vi "micro_Devices.vi"() -> ()   [LabVIEW 2014]
doc: "André Romero - 2023\nandretec@ifsc.usp.br\nIFSC - USP"
uses:
  Controller.ctl
  Thorlabs-Vector-Move/aptTec/Thorlabs-V2/Global Motors.vi
panel:
  out "Z ini":dbl
  out "Array Structures Ind":refnum<vi>[](array[refnum])
  in  "Tab Control":T1(tab)=enum."Cubes"
  in  "start-stop":bool
  in  "step size (mm)":dbl=10.0
  in  "Min   Z":bool
  in  "Max  Z":bool
  in  "Min":bool
  in  "Max":bool
  in  "Z (m/s)":dbl=50.0
  in  "XY (m/s)":dbl format="%#_5g"
  out "Motor Y":bool=TRUE
  out "Motor X":bool=TRUE
  out "Motor Z":bool=TRUE
  in  "Motor - Z":refnum<k7>(container)
  in  "Motor - Y":refnum<k7>(container)
  in  "Motor - X":refnum<k7>(container)
  out "current cube":i32
  out "current Layer":i32=1
  out "Total Progress (%)":u8(slide) caption="Layer Progress (%)" scale=0.0..25.0
  out "Layer Progress (%)":u8(slide)=100 scale=0.0..100.0
  in  "Line step size (mm)":dbl=1.0
  out "Lines Progress (%)":u8(slide)=42 scale=0.0..100.0
  in  "Stop Button":bool
  in  "Go Cubes":bool
  in  "Array of Structures":bool
  in  "Velocity (m/s)":dbl=50.0
  out "Layers":dbl=1.0
  in  "Delta Y (um)":dbl=50.0
  in  "Delta X (um)":dbl=50.0
  in  "Number of Lines":i32=2
  in  "Number of Columns":i32=5
  in  "Layer height (mm)":dbl=1.0
  in  "Height (mm)":dbl=1.0
  in  "Length (mm)":dbl=20.0
  in  "Width (mm)":dbl=20.0
  out "X ini":dbl
  out "Y ini":dbl
  in  "Initial position Z":bool=TRUE
  in  "Z offset (mm)":dbl=10.0
  in  "Z offset":bool
  in  "Motor - Z2":refnum<k7>(container)
  out "XY Graph":cluster{dbl[], dbl[]}(graph)
  in  "Go Test":bool
  in  "Density points":i32
  # "Velocity"
  # "Jog"
  # "mm"
  # "Z"
  # "Settings"
  # "Control"
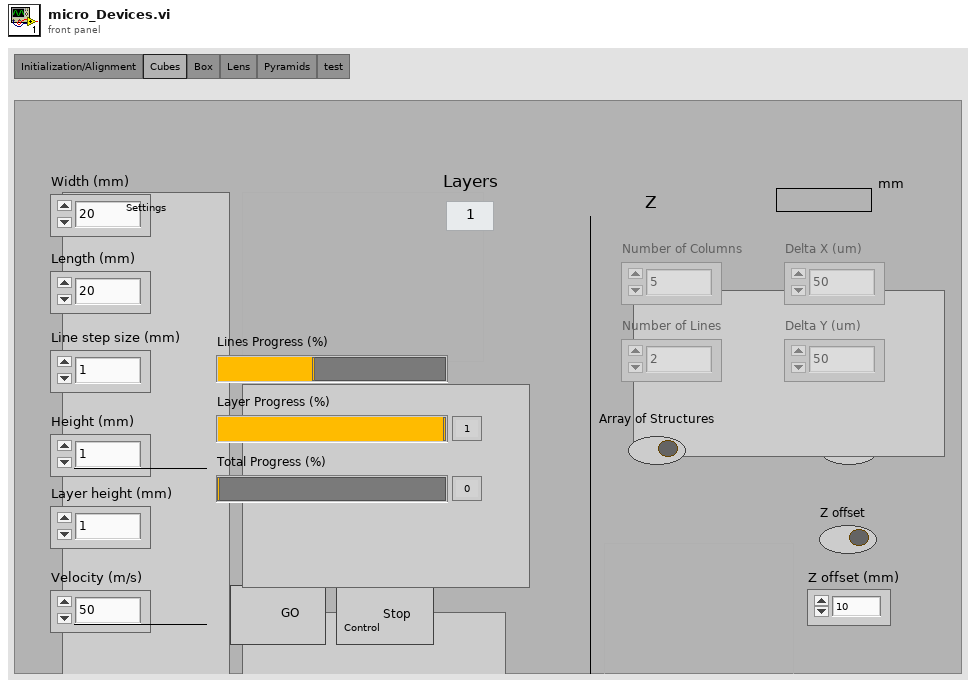
[diagram p1: front panel]
types:
  T1 = enum32{"Initialization/Alignment", "Cubes", "Box", "Lens", "Pyramids", "test"}
  T2 = typedef "Controller.ctl" = enum16{"Initialize", "Wait for Event", "Cubes", "Lens", "Box", "test tap"}
  T3 = typedef "eventvkey.ctl" = enum16{"ASCII", "Enter", "Return", "Shift", "Ctrl", "Alt", "Cmd", "Opt", "Caps", "NumLock", "Clear", "Break", "Up", "Down", "Left", "Right", "Insert", "Delete", "Home", "End", "PageUp", "PageDown", "Escape", "Help", "Pause", "ScrollLock", "F1", "F2", "F3", "F4", "F5", "F6", "F7", "F8", "F9", "F10", "F11", "F12", "F13", "F14", "F15", "F16", "F17", "F18", "F19", "F20", "F21", "F22", "F23", "F24", "Play", "VolumeUp", "VolumeDown", "Mute", "Two Byte Char"}
  T4 = enum8{"Enabled", "Disabled", "Disabled and Grayed Out"}
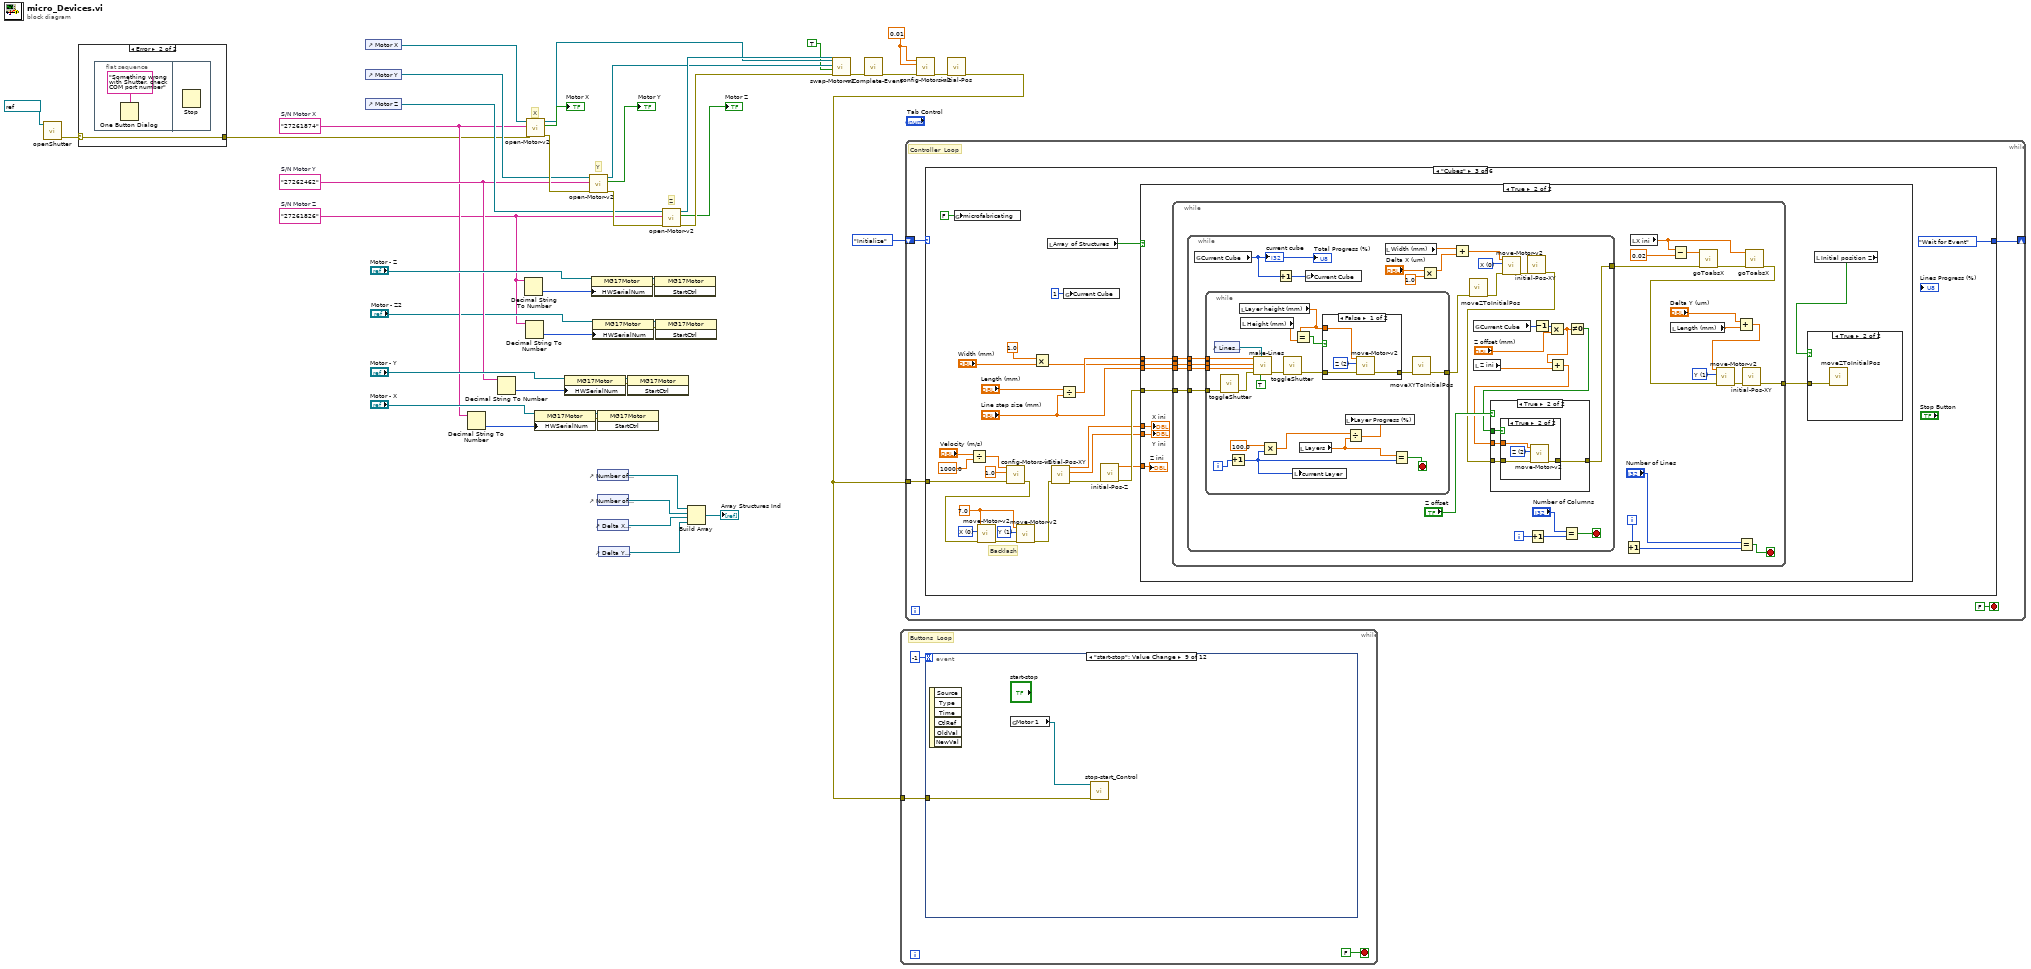
[diagram p0: block diagram]
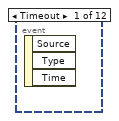
[diagram p3: hidden frame]
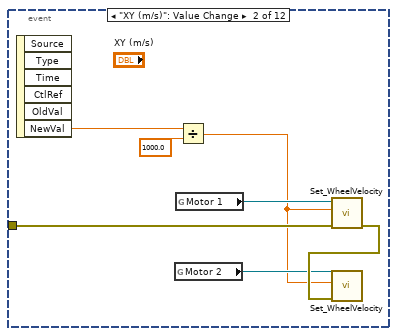
[diagram p4: hidden frame]
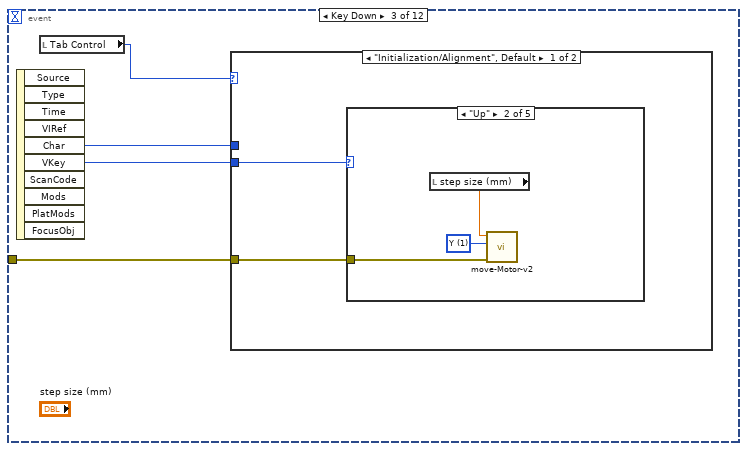
[diagram p5: hidden frame]
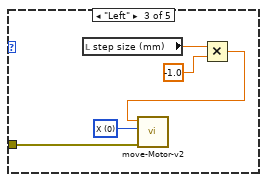
[diagram p7: hidden frame]
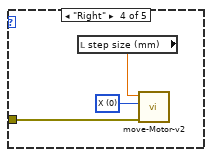
[diagram p8: hidden frame]
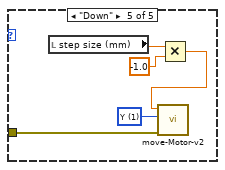
[diagram p9: hidden frame]
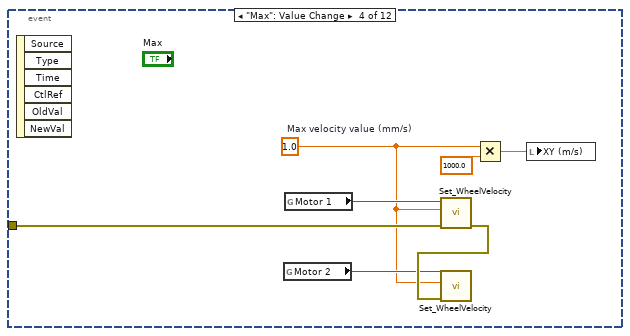
[diagram p11: hidden frame]
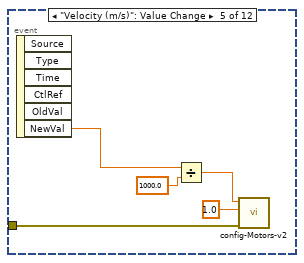
[diagram p12: hidden frame]
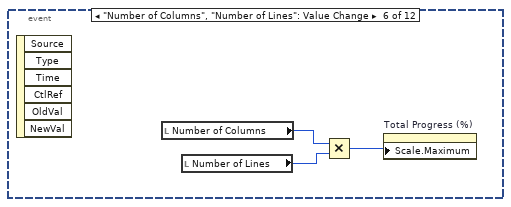
[diagram p13: hidden frame]
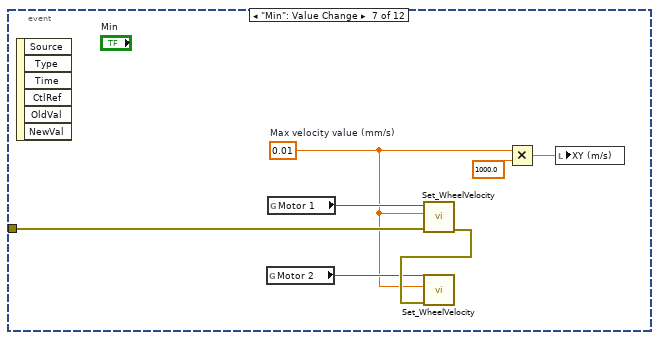
[diagram p14: hidden frame]
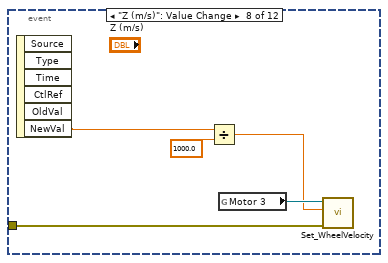
[diagram p15: hidden frame]
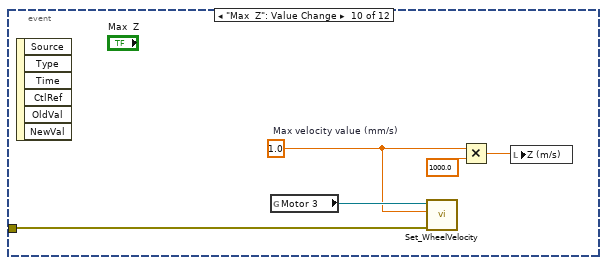
[diagram p16: hidden frame]
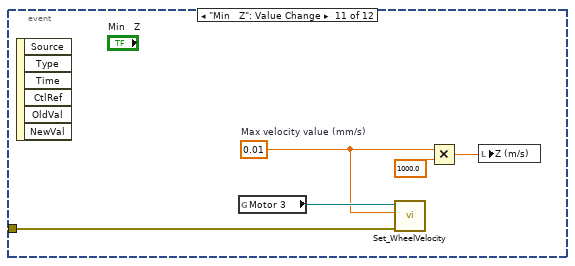
[diagram p17: hidden frame]
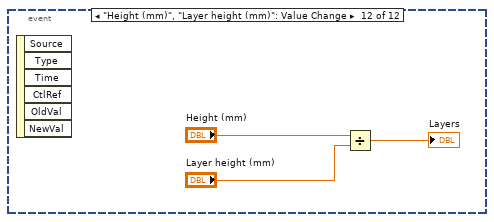
[diagram p18: hidden frame]
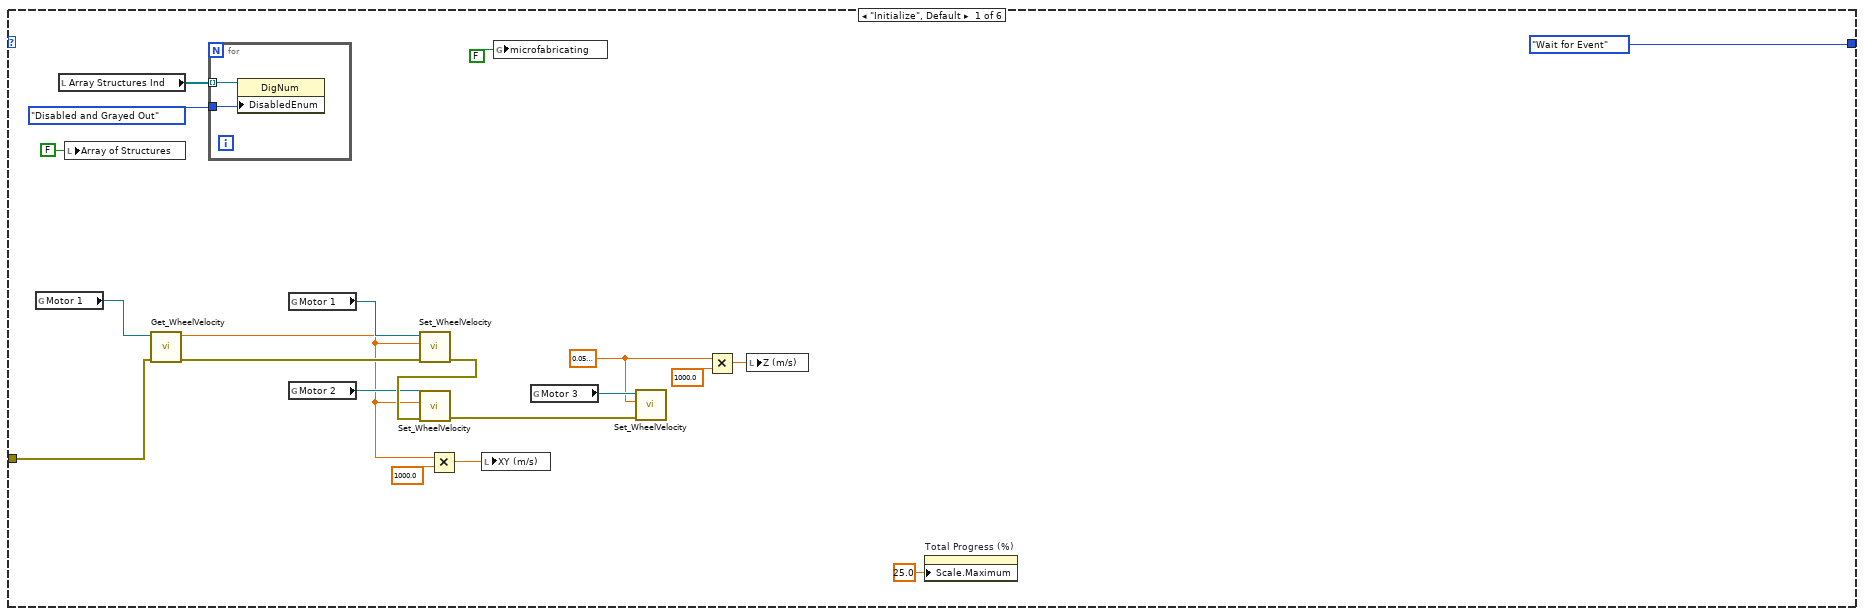
[diagram p19: hidden frame]
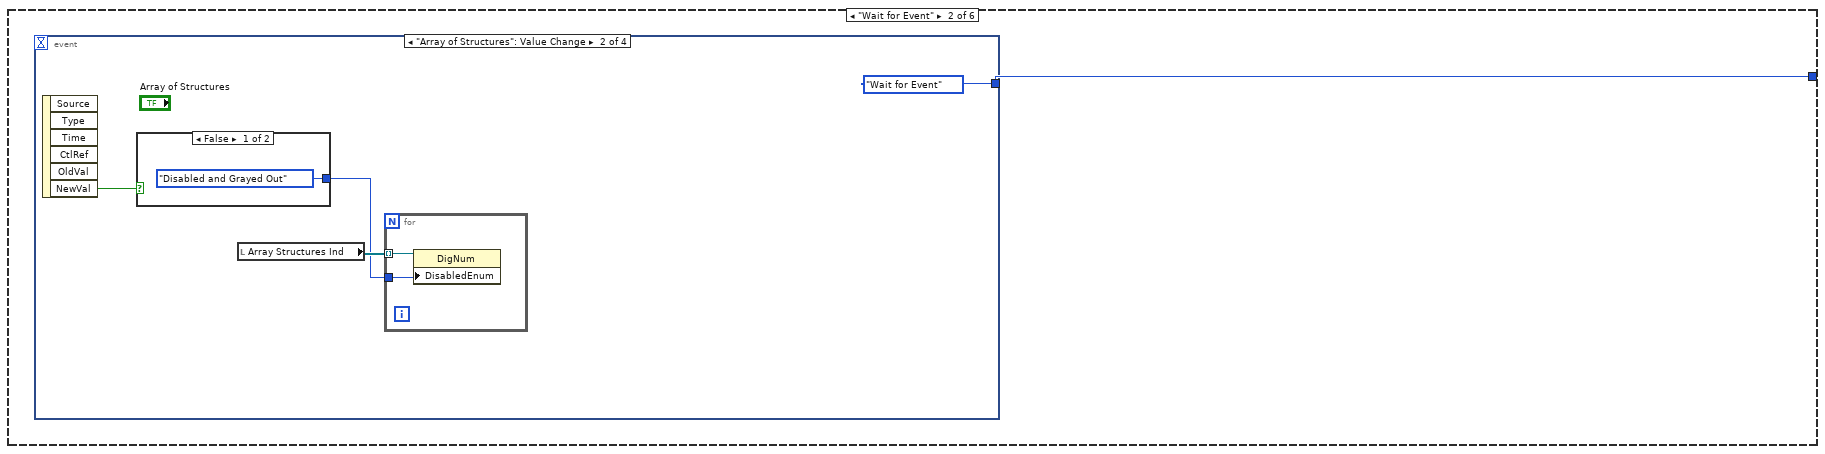
[diagram p20: hidden frame]
diagram:
  w29 = 0.01 ("Acc")
  w16 = "27262462"  # S/N Motor Y
  w15 = "27261874"  # S/N Motor X
  w1 = "27261826"  # S/N Motor Z
  # "X"
  # "Y"
  # "Z"
  n1 = call "openShutter.vi"("VISA Refnum in"=refnum<visa-resource-name> "COM3") -> ("error out"=w7:errorcluster)  [unwired: 9 in, 1 out]
  n2 = case shown="Error" w7 {
    selector: w7 -> [w47 w48]
    tunnel: [w47 w48] -> w6
    frame No Error {
    }
    frame Error {
      n3 = flat-sequence {
        frame #0 {
          n4 = One Button Dialog(message="Something wrong with Shutter, check COM port number") -> ()  [unwired: 1 in, 1 out]
        }
        frame #1 {
          n5 = Stop() -> ()  [unwired: 1 in]
        }
      }
    }
  }
  n6 = control-ref of="Motor X"() -> (w43:refnum<vi>)
  n7 = control-ref of="Motor Y"() -> (w42:refnum<vi>)
  n8 = control-ref of="Motor Z"() -> (w38:refnum<vi>)
  n9 = Decimal String To Number(string=w15) -> (number=w17:i32)  [unwired: 2 in, 1 out]
  n10 = Decimal String To Number(string=w16) -> (number=w21:i32)  [unwired: 2 in, 1 out]
  n11 = Decimal String To Number(string=w1) -> (number=w25:i32)  [unwired: 2 in, 1 out]
  n12 = Decimal String To Number(string=w1) -> (number=w2:i32)  [unwired: 2 in, 1 out]
  n13 = call "open-Motor-v2.vi"("Error In"=w6, "S/N Motor"=w15, "ref Boolean in"=w43) -> ("Error Out"=w46:errorcluster, "Motor Status"=→"Motor X":bool, "Refnum out"=w11:refnum<k7>)  [unwired: 6 in]
  n14 = property class="MG17Motor"(reference="Motor - X", "HWSerialNum"=w17) -> (reference out=w18:refnum<k7>, error out=w19:errorcluster)  [unwired: 1 in]
  n15 = property class="MG17Motor"(reference="Motor - Y", "HWSerialNum"=w21) -> (reference out=w22:refnum<k7>, error out=w23:errorcluster)  [unwired: 1 in]
  n16 = call "open-Motor-v2.vi"("Error In"=w46, "S/N Motor"=w16, "ref Boolean in"=w42) -> ("Error Out"=w40:errorcluster, "Motor Status"=→"Motor Y":bool, "Refnum out"=w10:refnum<k7>)  [unwired: 6 in]
  n17 = property class="MG17Motor"(reference="Motor - Z", "HWSerialNum"=w25) -> (reference out=w26:refnum<k7>, error out=w27:errorcluster)  [unwired: 1 in]
  n18 = property class="MG17Motor"(reference="Motor - Z2", "HWSerialNum"=w2) -> (reference out=w3:refnum<k7>, error out=w4:errorcluster)  [unwired: 1 in]
  n19 = invoke class="MG17Motor" method="StartCtrl"(reference=w18, error in=w19) -> ()  [unwired: 1 in, 3 out]
  n20 = control-ref of="Number of Lines"() -> (w34:refnum<vi>)
  n21 = control-ref of="Number of Columns"() -> (w33:refnum<vi>)
  n22 = control-ref of="Delta X (um)"() -> (w32:refnum<vi>)
  n23 = control-ref of="Delta Y (um)"() -> (w31:refnum<vi>)
  n24 = invoke class="MG17Motor" method="StartCtrl"(reference=w22, error in=w23) -> ()  [unwired: 1 in, 3 out]
  n25 = invoke class="MG17Motor" method="StartCtrl"(reference=w26, error in=w27) -> ()  [unwired: 1 in, 3 out]
  n26 = invoke class="MG17Motor" method="StartCtrl"(reference=w3, error in=w4) -> ()  [unwired: 1 in, 3 out]
  n27 = call "open-Motor-v2.vi"("Error In"=w40, "S/N Motor"=w1, "ref Boolean in"=w38) -> ("Error Out"=w39:errorcluster, "Motor Status"=→"Motor Z":bool, "Refnum out"=w36:refnum<k7>)  [unwired: 6 in]
  n28 = Build Array(w34, w33, w32, w31) -> (→"Array Structures Ind":refnum<vi>[])
  n29 = call "swap-Motor-v2.vi"("Refnum in M3"=w36, "error in (no error)"=w39, "Swap motor"=TRUE, "Refnum in M2"=w10, "Refnum in M1"=w11) -> ("error out"=w14:errorcluster)  [unwired: 6 in]
  n30 = call "mComplete-Event.vi"("Error In"=w14) -> ("Error Out"=w13:errorcluster)  [unwired: 10 in]
  n31 = call "config-Motors-v2.vi"("error in"=w13, "Acc"=w29, "Velocity"=w29) -> ("error out"=w41:errorcluster)  [unwired: 8 in]
  n32 = call "initial-Pos.vi"("error in (no error)"=w41) -> ("error out"=w12:errorcluster)  [unwired: 10 in]
  n33 = while {
    tunnel: w12 -> [w51]
    stop <- FALSE stop-if-true
    # "Buttons  Loop"
    n34 = event shown="[8] \"start-stop\": Value Change" {
      selector: _ -> [_ _ _ _ _ _ _ _ _ _ _ _]
      dyn-events: _ -> [_ _ _ _ _ _ _ _ _ _ _ _]
      timeout: -1 -> [_ _ _ _ _ _ _ _ _ _ _ _]
      tunnel: w51 -> [_ w58 w60 w85 w89 _ w100 w104 w110 w111 w116 _]
      event Timeout {
        n35 = event-data() -> ()  [unwired: 1 in, 3 out]
      }
      event "XY (m/s)": Value Change {
        n36 = event-data() -> ("NewVal"=w55:dbl)  [unwired: 1 in, 5 out]
        n37 = global read "Global Motors.vi" "Motor 2"() -> (w56:refnum<k7>)
        n38 = global read "Global Motors.vi" "Motor 1"() -> (w59:refnum<k7>)
        n39 = Divide(x=w55, y=1000.0) -> (x/y=w54:dbl)
        n40 = call "Set_WheelVelocity.vi"("error in"=w58, "fWheelVel"=w54, "MG17Motor in"=w59) -> ("error out"=w57:errorcluster)  [unwired: 8 in]
        n41 = call "Set_WheelVelocity.vi"("error in"=w57, "fWheelVel"=w54, "MG17Motor in"=w56) -> ()  [unwired: 8 in, 1 out]
      }
      event Key Down {
        n42 = event-data() -> ("Char"=w62:i16, "VKey"=w61:T3)  [unwired: 1 in, 8 out]
        n43 = local read "Tab Control"() -> (w63:T1)
        n44 = case shown="\"Initialization/Alignment\", Default" w63 {
          tunnel: w62 -> [_ _]
          tunnel: w61 -> [w65 _]
          tunnel: w60 -> [w64 _]
          frame "Initialization/Alignment", Default {
            n45 = case shown="\"Up\"" w65 {
              tunnel: w64 -> [_ w68 w73 w76 w80]
              frame "ASCII", Default {
              }
              frame "Up" {
                w67 = u16 1 items=["X", "Y", "Z"] ("Axis")
                n46 = local read "step size (mm)"() -> (w66:dbl)
                n47 = call "move-Motor-v2.vi"("error in"=w68, "Axis"=w67, "Distance (um)"=w66) -> ()  [unwired: 8 in, 1 out]
              }
              frame "Left" {
                w72 = u16 0 items=["X", "Y", "Z"] ("Axis")
                n48 = local read "step size (mm)"() -> (w71:dbl)
                n49 = Multiply(x=w71, y=-1.0) -> (x*y=w69:dbl)
                n50 = call "move-Motor-v2.vi"("error in"=w73, "Axis"=w72, "Distance (um)"=w69) -> ()  [unwired: 8 in, 1 out]
              }
              frame "Right" {
                w75 = u16 0 items=["X", "Y", "Z"] ("Axis")
                n51 = local read "step size (mm)"() -> (w74:dbl)
                n52 = call "move-Motor-v2.vi"("error in"=w76, "Axis"=w75, "Distance (um)"=w74) -> ()  [unwired: 8 in, 1 out]
              }
              frame "Down" {
                w81 = u16 1 items=["X", "Y", "Z"] ("Axis")
                n53 = local read "step size (mm)"() -> (w79:dbl)
                n54 = Multiply(x=w79, y=-1.0) -> (x*y=w77:dbl)
                n55 = call "move-Motor-v2.vi"("error in"=w80, "Axis"=w81, "Distance (um)"=w77) -> ()  [unwired: 8 in, 1 out]
              }
            }
          }
          frame "Cubes" {
          }
        }
      }
      event "Max": Value Change {
        w83 = 1.0  # Max velocity value (mm/s)
        n56 = event-data() -> ()  [unwired: 1 in, 6 out]
        n57 = global read "Global Motors.vi" "Motor 2"() -> (w86:refnum<k7>)
        n58 = global read "Global Motors.vi" "Motor 1"() -> (w88:refnum<k7>)
        n59 = call "Set_WheelVelocity.vi"("error in"=w85, "fWheelVel"=w83, "MG17Motor in"=w88) -> ("error out"=w87:errorcluster)  [unwired: 8 in]
        n60 = call "Set_WheelVelocity.vi"("error in"=w87, "fWheelVel"=w83, "MG17Motor in"=w86) -> ()  [unwired: 8 in, 1 out]
        n61 = Multiply(x=w83, y=1000.0) -> (x*y=w82:dbl)
        n62 = local write "XY (m/s)"(w82) -> ()
      }
      event "Velocity (m/s)": Value Change {
        n63 = event-data() -> ("NewVal"=w93:dbl)  [unwired: 1 in, 5 out]
        n64 = Divide(x=w93, y=1000.0) -> (x/y=w91:dbl)
        n65 = call "config-Motors-v2.vi"("error in"=w89, "Acc"=1.0, "Velocity"=w91) -> ()  [unwired: 8 in, 1 out]
      }
      event "Number of Columns", "Number of Lines": Value Change {
        n66 = event-data() -> ()  [unwired: 1 in, 6 out]
        n67 = local read "Number of Columns"() -> (w95:i32)
        n68 = local read "Number of Lines"() -> (w96:i32)
        n69 = Multiply(x=w95, y=w96) -> (x*y=w94:i32)
        n70 = property on="Total Progress (%)" class="Slide (strict)"("Scale.Maximum"=w94) -> ()  [unwired: 2 in, 2 out]
      }
      event "Min": Value Change {
        w98 = 0.01  # Max velocity value (mm/s)
        n71 = event-data() -> ()  [unwired: 1 in, 6 out]
        n72 = global read "Global Motors.vi" "Motor 2"() -> (w101:refnum<k7>)
        n73 = global read "Global Motors.vi" "Motor 1"() -> (w103:refnum<k7>)
        n74 = call "Set_WheelVelocity.vi"("error in"=w100, "fWheelVel"=w98, "MG17Motor in"=w103) -> ("error out"=w102:errorcluster)  [unwired: 8 in]
        n75 = call "Set_WheelVelocity.vi"("error in"=w102, "fWheelVel"=w98, "MG17Motor in"=w101) -> ()  [unwired: 8 in, 1 out]
        n76 = Multiply(x=w98, y=1000.0) -> (x*y=w97:dbl)
        n77 = local write "XY (m/s)"(w97) -> ()
      }
      event "Z (m/s)": Value Change {
        n78 = event-data() -> ("NewVal"=w107:dbl)  [unwired: 1 in, 5 out]
        n79 = Divide(x=w107, y=1000.0) -> (x/y=w105:dbl)
        n80 = global read "Global Motors.vi" "Motor 3"() -> (w106:refnum<k7>)
        n81 = call "Set_WheelVelocity.vi"("error in"=w104, "fWheelVel"=w105, "MG17Motor in"=w106) -> ()  [unwired: 8 in, 1 out]
      }
      event "start-stop": Value Change {
        n82 = event-data() -> ()  [unwired: 1 in, 6 out]
        n83 = global read "Global Motors.vi" "Motor 1"() -> (w109:refnum<k7>)
        n84 = call "stop-start_Control.vi"("error in (no error)"=w110, "Automation Refnum in"=w109) -> ()  [unwired: 8 in, 2 out]
      }
      event "Max  Z": Value Change {
        w113 = 1.0  # Max velocity value (mm/s)
        n85 = event-data() -> ()  [unwired: 1 in, 6 out]
        n86 = global read "Global Motors.vi" "Motor 3"() -> (w115:refnum<k7>)
        n87 = call "Set_WheelVelocity.vi"("error in"=w111, "fWheelVel"=w113, "MG17Motor in"=w115) -> ()  [unwired: 8 in, 1 out]
        n88 = Multiply(x=w113, y=1000.0) -> (x*y=w112:dbl)
        n89 = local write "Z (m/s)"(w112) -> ()
      }
      event "Min   Z": Value Change {
        w118 = 0.01  # Max velocity value (mm/s)
        n90 = event-data() -> ()  [unwired: 1 in, 6 out]
        n91 = global read "Global Motors.vi" "Motor 3"() -> (w120:refnum<k7>)
        n92 = call "Set_WheelVelocity.vi"("error in"=w116, "fWheelVel"=w118, "MG17Motor in"=w120) -> ()  [unwired: 8 in, 1 out]
        n93 = Multiply(x=w118, y=1000.0) -> (x*y=w117:dbl)
        n94 = local write "Z (m/s)"(w117) -> ()
      }
      event "Height (mm)", "Layer height (mm)": Value Change {
        n95 = event-data() -> ()  [unwired: 1 in, 6 out]
        n96 = Divide(x="Height (mm)", y="Layer height (mm)") -> (x/y=→"Layers":dbl)
      }
    }
  }
  n97 = while {
    shift-right: [w125] -> _
    shift-left: Controller."Initialize" -> [w126]
    tunnel: w12 -> [w124]
    stop <- FALSE stop-if-true
    # "Controller  Loop"
    n98 = case shown="\"Cubes\"" w126 {
      tunnel: [Controller."Wait for Event" w150 Controller."Wait for Event" Controller."Wait for Event" Controller."Wait for Event" Controller."Wait for Event"] -> w125
      tunnel: w124 -> [w129 _ w187 _ _ w325]
      frame "Initialize", Default {
        w133 = sgl 0.05 ("fWheelVel")
        n99 = global read "Global Motors.vi" "Motor 1"() -> (w143:refnum<k7>)
        n100 = local read "Array Structures Ind"() -> (w145:refnum<vi>[])
        n101 = local write "Array of Structures"(FALSE ("Array of Structures")) -> ()
        n102 = call "Get_WheelVelocity.vi"("error in"=w129, "MG17Motor in"=w143) -> ("error out"=w139:errorcluster, "pfWheelVel"=w138:sgl)  [unwired: 8 in]
        n103 = for {
          tunnel: T4."Disabled and Grayed Out" ("Disabled") -> [w149]
          tunnel: w145 -> [w148] mode=indexing
          n104 = property class="DigNum"(reference=w148, "DisabledEnum"=w149) -> ()  [unwired: 1 in, 2 out]
        }
        n105 = global read "Global Motors.vi" "Motor 1"() -> (w142:refnum<k7>)
        n106 = global read "Global Motors.vi" "Motor 2"() -> (w140:refnum<k7>)
        n107 = call "Set_WheelVelocity.vi"("error in"=w139, "fWheelVel"=w138, "MG17Motor in"=w142) -> ("error out"=w141:errorcluster)  [unwired: 8 in]
        n108 = call "Set_WheelVelocity.vi"("error in"=w141, "fWheelVel"=w138, "MG17Motor in"=w140) -> ("error out"=w135:errorcluster)  [unwired: 8 in]
        n109 = Multiply(x=w138, y=sgl 1000.0) -> (x*y=w137:sgl)
        n110 = local write "XY (m/s)"(w137) -> ()
        n111 = global write "Global micro_Devices.vi" "microfabricating"(FALSE ("microfabricating")) -> ()
        n112 = global read "Global Motors.vi" "Motor 3"() -> (w134:refnum<k7>)
        n113 = call "Set_WheelVelocity.vi"("error in"=w135, "fWheelVel"=w133, "MG17Motor in"=w134) -> ()  [unwired: 8 in, 1 out]
        n114 = Multiply(x=w133, y=sgl 1000.0) -> (x*y=w132:sgl)
        n115 = local write "Z (m/s)"(w132) -> ()
        n116 = property on="Total Progress (%)" class="Slide (strict)"("Scale.Maximum"=25.0 ("Scale.Range:Maximum")) -> ()  [unwired: 2 in, 2 out]
      }
      frame "Wait for Event" {
        n117 = event shown="[1] \"Array of Structures\": Value Change" {
          selector: _ -> [_ _ _ _]
          dyn-events: _ -> [_ _ _ _]
          timeout: _ -> [_ _ _ _]
          tunnel: [Controller."Wait for Event" Controller."Wait for Event" w160 w164] -> w150
          event Timeout {
            n118 = event-data() -> ()  [unwired: 1 in, 3 out]
          }
          event "Array of Structures": Value Change {
            n119 = event-data() -> ("NewVal"=w153:bool)  [unwired: 1 in, 5 out]
            n120 = case shown="False" w153 {
              tunnel: [T4."Disabled and Grayed Out" ("Disabled") T4."Enabled" ("Disabled")] -> w154
              frame False {
              }
              frame True {
              }
            }
            n121 = local read "Array Structures Ind"() -> (w155:refnum<vi>[])
            n122 = for {
              tunnel: w154 -> [w157]
              tunnel: w155 -> [w156] mode=indexing
              n123 = property class="DigNum"(reference=w156, "DisabledEnum"=w157) -> ()  [unwired: 1 in, 2 out]
            }
          }
          event "Go Cubes": Value Change {
            n124 = event-data() -> ()  [unwired: 1 in, 6 out]
            n125 = global read "Global micro_Devices.vi" "microfabricating"() -> (w161:bool)
            n126 = case shown="False" w161 {
              tunnel: [Controller."Cubes" Controller."Wait for Event"] -> w160
              frame False {
              }
              frame True {
              }
            }
          }
          event "Go Test": Value Change {
            n127 = event-data() -> ()  [unwired: 1 in, 6 out]
            n128 = global read "Global micro_Devices.vi" "microfabricating"() -> (w165:bool)
            n129 = case shown="False" w165 {
              tunnel: [Controller."test tap" Controller."Wait for Event"] -> w164
              frame False {
              }
              frame True {
              }
            }
          }
        }
      }
      frame "Cubes" {
        w174 = u16 1 items=["X", "Y", "Z"] ("Axis")
        w173 = 7.0 ("Distance (um)")
        w176 = u16 0 items=["X", "Y", "Z"] ("Axis")
        # "Backlash"
        n130 = global write "Global micro_Devices.vi" "microfabricating"(FALSE ("microfabricating")) -> ()
        n131 = Divide(x="Velocity (m/s)", y=1000.0) -> (x/y=w178:dbl)
        n132 = call "config-Motors-v2.vi"("error in"=w187, "Acc"=1.0, "Velocity"=w178) -> ("error out"=w172:errorcluster)  [unwired: 8 in]
        n133 = call "move-Motor-v2.vi"("error in"=w172, "Axis"=w176, "Distance (um)"=w173) -> ("error out"=w175:errorcluster)  [unwired: 8 in]
        n134 = call "move-Motor-v2.vi"("error in"=w175, "Axis"=w174, "Distance (um)"=w173) -> ("error out"=w171:errorcluster)  [unwired: 8 in]
        n135 = Multiply(x=1.0, y="Width (mm)") -> (x*y=w169:dbl)
        n136 = local read "Array of Structures"() -> (w182:bool)
        n137 = call "initial-Pos-XY.vi"("error in (no error)"=w171) -> ("error out"=w184:errorcluster, "Y position"=w180:dbl, "X position"=w181:dbl)  [unwired: 8 in]
        n138 = Divide(x="Length (mm)", y="Line step size (mm)") -> (x/y=w189:dbl)
        n139 = global write "Global micro_Devices.vi" "Current Cube"(1 ("Current Cube")) -> ()
        n140 = call "initial-Pos-Z.vi"("error in (no error)"=w184) -> ("error out"=w183:errorcluster, "Z position"=w179:dbl)  [unwired: 9 in]
        n141 = case shown="True" w182 {
          tunnel: w169 -> [w199 w234]
          tunnel: w189 -> [w198 w235]
          tunnel: "Line step size (mm)" -> [w197 w233]
          tunnel: w183 -> [w196 w232]
          tunnel: w181 -> [_ w231]
          tunnel: w180 -> [_ w230]
          tunnel: w179 -> [_ w229]
          frame False {
            n142 = while {
              tunnel: w199 -> [w221]
              tunnel: w198 -> [w220]
              tunnel: w197 -> [w219]
              tunnel: w196 -> [w217]
              tunnel: [w210] -> w195
              i -> [w213]
              stop <- w212 stop-if-true
              n143 = call "toggleShutter.vi"("Error In"=w217) -> ("error out"=w216:errorcluster)  [unwired: 9 in]
              n144 = Increment(x=w213) -> (x+1=w208:i32)
              "current Layer" <- w208
              n145 = local read "Layer height (mm)"() -> (w204:dbl)
              n146 = local read "Height (mm)"() -> (w203:dbl)
              n147 = control-ref of="Lines Progress (%)"() -> (w218:refnum<vi>)
              n148 = Multiply(x=100.0, y=w208) -> (x*y=w207:dbl)
              n149 = call "make-Lines.vi"("Shutter off between lines"=TRUE, "Slide in"=w218, "error in"=w216, "d (um)"=w219, "L (um)"=w221, "N Lines"=w220) -> ("error out"=w215:errorcluster)  [unwired: 4 in, 1 out]
              n150 = call "toggleShutter.vi"("Error In"=w215) -> ("error out"=w214:errorcluster)  [unwired: 9 in]
              n151 = local read "Layers"() -> (w206:dbl)
              n152 = Equal?(x=w203, y=w204) -> (x = y?=w202:bool)
              n153 = Divide(x=w207, y=w206) -> (x/y=→"Layer Progress (%)":dbl)
              n154 = case shown="False" w202 {
                tunnel: w214 -> [w224 w226]
                tunnel: [w223 w226] -> w211
                tunnel: w204 -> [w222 _]
                frame False {
                  w225 = u16 2 items=["X", "Y", "Z"] ("Axis")
                  n155 = call "move-Motor-v2.vi"("error in"=w224, "Axis"=w225, "Distance (um)"=w222) -> ("error out"=w223:errorcluster)  [unwired: 8 in]
                }
                frame True {
                }
              }
              n156 = Equal?(x=w206, y=w208) -> (x = y?=w212:bool)
              n157 = call "moveXYToInitialPos.vi"("error in"=w211) -> ("error out"=w210:errorcluster)  [unwired: 10 in]
            }
            n158 = case shown="True" "Initial position Z" {
              tunnel: w195 -> [_ w200]
              frame False {
              }
              frame True {
                n159 = call "moveZToInitialPos.vi"("error in"=w200) -> ()  [unwired: 10 in, 1 out]
              }
            }
          }
          frame True {
            n160 = while {
              tunnel: w235 -> [w256]
              tunnel: w234 -> [w255]
              tunnel: w233 -> [w254]
              tunnel: w232 -> [w253]
              tunnel: [w237] -> w227
              i -> [w250]
              stop <- w249 stop-if-true
              w248 = u16 1 items=["X", "Y", "Z"] ("Axis")
              n161 = while {
                tunnel: w256 -> [w285]
                tunnel: w255 -> [w284]
                tunnel: w254 -> [w283]
                tunnel: w253 -> [w282]
                tunnel: [w265] -> w238
                i -> [w275]
                stop <- w273 stop-if-true
                w280 = u16 0 items=["X", "Y", "Z"] ("Axis")
                n162 = global read "Global micro_Devices.vi" "Current Cube"() -> (w257:i32)
                "current cube" <- w257
                "Total Progress (%)" <- w257
                n163 = while {
                  tunnel: w285 -> [w313]
                  tunnel: w284 -> [w312]
                  tunnel: w283 -> [w311]
                  tunnel: w282 -> [w310]
                  tunnel: [w308] -> w281
                  i -> [w303]
                  stop <- w302 stop-if-true
                  n164 = control-ref of="Lines Progress (%)"() -> (w301:refnum<vi>)
                  n165 = call "toggleShutter.vi"("Error In"=w310) -> ("error out"=w309:errorcluster)  [unwired: 9 in]
                  n166 = Increment(x=w303) -> (x+1=w300:i32)
                  n167 = local read "Layer height (mm)"() -> (w298:dbl)
                  n168 = local read "Height (mm)"() -> (w297:dbl)
                  n169 = call "make-Lines.vi"("Shutter off between lines"=TRUE, "Slide in"=w301, "error in"=w309, "d (um)"=w311, "L (um)"=w312, "N Lines"=w313) -> ("error out"=w316:errorcluster)  [unwired: 4 in, 1 out]
                  n170 = Multiply(x=100.0, y=w300) -> (x*y=w305:dbl)
                  n171 = call "toggleShutter.vi"("Error In"=w316) -> ("error out"=w315:errorcluster)  [unwired: 9 in]
                  n172 = local write "current Layer"(w300) -> ()
                  n173 = Equal?(x=w298, y=w297) -> (x = y?=w299:bool)
                  n174 = local read "Layers"() -> (w306:dbl)
                  n175 = case shown="False" w299 {
                    tunnel: w315 -> [w319 w321]
                    tunnel: [w318 w321] -> w314
                    tunnel: w298 -> [w317 _]
                    frame False {
                      w320 = u16 2 items=["X", "Y", "Z"] ("Axis")
                      n176 = call "move-Motor-v2.vi"("error in"=w319, "Axis"=w320, "Distance (um)"=w317) -> ("error out"=w318:errorcluster)  [unwired: 8 in]
                    }
                    frame True {
                    }
                  }
                  n177 = Divide(x=w305, y=w306) -> (x/y=w304:dbl)
                  n178 = local write "Layer Progress (%)"(w304) -> ()
                  n179 = Equal?(x=w306, y=w300) -> (x = y?=w302:bool)
                  n180 = call "moveXYToInitialPos.vi"("error in"=w314) -> ("error out"=w308:errorcluster)  [unwired: 10 in]
                }
                n181 = Increment(x=w257) -> (x+1=w270:i32)
                n182 = global write "Global micro_Devices.vi" "Current Cube"(w270) -> ()
                n183 = local read "Width (mm)"() -> (w278:dbl)
                n184 = Multiply(x="Delta X (um)", y=1.0) -> (x*y=w269:dbl)
                n185 = Add(x=w278, y=w269) -> (x+y=w276:dbl)
                n186 = call "moveZToInitialPos.vi"("error in"=w281) -> ("error out"=w279:errorcluster)  [unwired: 10 in]
                n187 = global read "Global micro_Devices.vi" "Current Cube"() -> (w262:i32)
                n188 = local read "Z ini"() -> (w261:dbl)
                n189 = call "move-Motor-v2.vi"("error in"=w279, "Axis"=w280, "Distance (um)"=w276) -> ("error out"=w272:errorcluster)  [unwired: 8 in]
                n190 = call "initial-Pos-XY.vi"("error in (no error)"=w272) -> ("error out"=w266:errorcluster)  [unwired: 8 in, 2 out]
                n191 = Increment(x=w275) -> (x+1=w274:i32)
                n192 = Decrement(x=w262) -> (x-1=w263:i32)
                n193 = Multiply(x=w263, y="Z offset (mm)") -> (x*y=w260:dbl)
                n194 = Add(x=w260, y=w261) -> (x+y=w258:dbl)
                n195 = Equal?(x="Number of Columns", y=w274) -> (x = y?=w273:bool)
                n196 = Not Equal To 0?(x=w260) -> (x != 0?=w259:bool)
                n197 = case shown="True" "Z offset" {
                  tunnel: w266 -> [w286 w290]
                  tunnel: [w286 w289] -> w265
                  tunnel: w259 -> [_ w288]
                  tunnel: w258 -> [_ w287]
                  frame False {
                  }
                  frame True {
                    n198 = case shown="True" w288 {
                      tunnel: w290 -> [w291 w294]
                      tunnel: [w291 w293] -> w289
                      tunnel: w287 -> [_ w292]
                      frame False {
                      }
                      frame True {
                        w295 = u16 2 items=["X", "Y", "Z"] ("Axis")
                        n199 = call "move-Motor-v2.vi"("error in"=w294, "Axis"=w295, "Distance (um)"=w292) -> ("error out"=w293:errorcluster)  [unwired: 8 in]
                      }
                    }
                  }
                }
              }
              n200 = Increment(x=w250) -> (x+1=w244:i32)
              n201 = local read "X ini"() -> (w240:dbl)
              n202 = local read "Length (mm)"() -> (w251:dbl)
              n203 = Subtract(x=w240, y=0.02 ("x")) -> (x-y=w243:dbl)
              n204 = call "goToabsX.vi"("error in"=w238, "X position"=w243) -> ("error out"=w241:errorcluster)  [unwired: 9 in]
              n205 = Add(x="Delta Y (um)", y=w251) -> (x+y=w247:dbl)
              n206 = Equal?(x="Number of Lines", y=w244) -> (x = y?=w249:bool)
              n207 = call "goToabsX.vi"("error in"=w241, "X position"=w240) -> ("error out"=w239:errorcluster)  [unwired: 9 in]
              n208 = call "move-Motor-v2.vi"("error in"=w239, "Axis"=w248, "Distance (um)"=w247) -> ("error out"=w246:errorcluster)  [unwired: 8 in]
              n209 = call "initial-Pos-XY.vi"("error in (no error)"=w246) -> ("error out"=w237:errorcluster)  [unwired: 8 in, 2 out]
            }
            n210 = local read "Initial position Z"() -> (w228:bool)
            n211 = case shown="True" w228 {
              tunnel: w227 -> [_ w236]
              frame False {
              }
              frame True {
                n212 = call "moveZToInitialPos.vi"("error in"=w236) -> ()  [unwired: 10 in, 1 out]
              }
            }
            "X ini" <- w231
            "Y ini" <- w230
            "Z ini" <- w229
          }
        }
      }
      frame "Lens" {
      }
      frame "Box" {
      }
      frame "test tap" {
        n213 = disable-structure shown="Enabled" {
          disable-tunnel: w325 -> [w330 w334]
          disable-tunnel: [w329 w334] -> w324
          frame Disabled {
            w332 = u16 1 items=["X", "Y", "Z"] ("Axis")
            w333 = u16 0 items=["X", "Y", "Z"] ("Axis")
            w331 = 10.0 ("Distance (um)")
            n214 = call "move-Motor-v2.vi"("error in"=w330, "Axis"=w332, "Distance (um)"=w331) -> ("error out"=w328:errorcluster)  [unwired: 8 in]
            n215 = call "move-Motor-v2.vi"("error in"=w328, "Axis"=w333, "Distance (um)"=w331) -> ("error out"=w329:errorcluster)  [unwired: 8 in]
          }
          frame Enabled {
          }
        }
        n216 = call "get-Position-v2.vi"("error in (no error)"=w324) -> ()  [unwired: 7 in, 4 out]
        n217 = for {
          N: "Density points" -> [w345]
          i -> [w343]
          n218 = Divide(x=6.283185307179586, y=w345) -> (x/y=w344:dbl)
          n219 = Multiply(x=w344, y=w343) -> (x*y=w342:dbl)
          n220 = Sine & Cosine(0:w342) -> (1:w340:dbl, 2:w335:dbl)
          n221 = feedback #1() -> (w339:dbl[])  [unwired: 1 in]
          n222 = Build Array (concatenate)(w339, w335) -> (w336:dbl[])
          n223 = feedback-in #1(w336) -> ()
          n224 = feedback #2() -> (w341:dbl[])  [unwired: 1 in]
          n225 = Build Array (concatenate)(w341, w340) -> (w337:dbl[])
          n226 = feedback-in #2(w337) -> ()
          n227 = Bundle(w337, w336) -> (→"XY Graph":cluster{dbl[], dbl[]})  [unwired: 1 in]
        }
      }
    }
  }
